vi "CMD tasklist.vi"(8 "error in":errorcluster, 11 "PID":string) -> (0 "error out":errorcluster, 1 "output":string, 2 "tasklist command":string, 3 "Finished":bool)   [LabVIEW 2019, in "PostBuildSupport.lvclass"]
uses:
  PostBuildSupport.lvclass
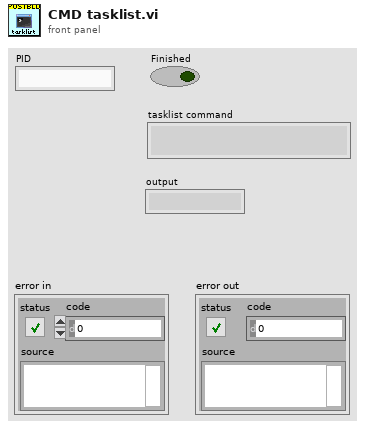
[diagram p1: front panel]
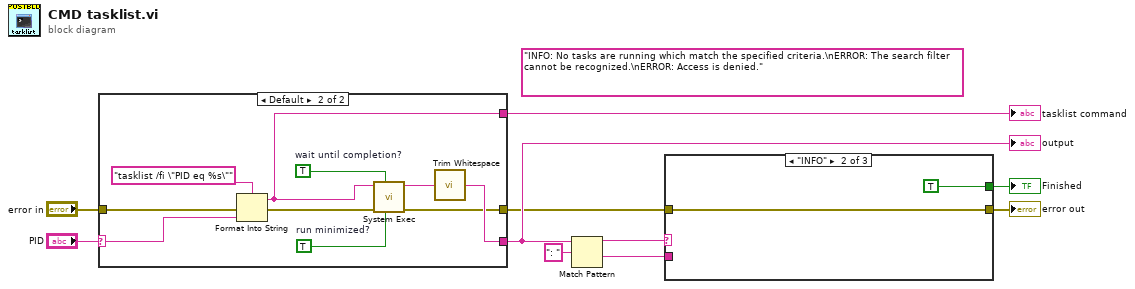
[diagram p0: block diagram]
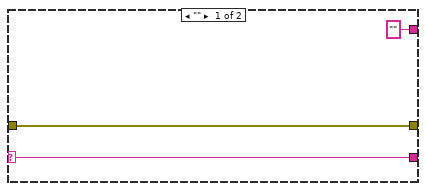
[diagram p2: hidden frame]
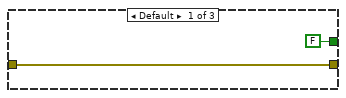
[diagram p3: hidden frame]
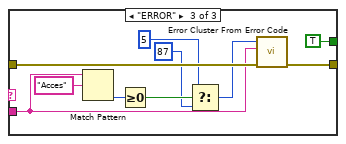
[diagram p4: hidden frame]
diagram:
  (unwired) "INFO: No tasks are running which match the specified criteria.\nERROR: The search filter cannot be recognized.\nERROR: Access is denied." ("x")
  n1 = case shown="Default" "PID" {
    selector: "PID" -> [w13 w20]
    tunnel: [w13 w16] -> w7
    tunnel: "error in" -> [w11 w18]
    tunnel: ["" w15] -> w8
    tunnel: [w11 w14] -> w4
    frame "" {
    }
    frame Default {
      w23 = TRUE  # run minimized?
      w22 = TRUE  # wait until completion?
      n2 = Format Into String(format string="tasklist /fi \"PID eq %s\"" ("command line"), error in=w18, w20) -> (resulting string=w15:string, error out=w17:errorcluster)  [unwired: 1 in]
      n3 = call <vilib>:"System Exec.vi"("run minimized? (F)"=w23, "wait until completion? (T)"=w22, "error in (no error)"=w17, "command line"=w15) -> ("error out"=w14:errorcluster, "standard output"=w19:string)  [unwired: 4 in, 2 out]
      n4 = call <vilib>:"Trim Whitespace.vi"("string"=w19) -> ("trimmed string"=w16:string)  [unwired: 1 in]
    }
  }
  "output" <- w7
  "tasklist command" <- w8
  n5 = Match Pattern(string=w7, regular expression=": ") -> (before substring=w5:string, after substring=w3:string)  [unwired: 1 in, 2 out]
  n6 = case shown="\"INFO\"" w5 {
    tunnel: w4 -> [w25 w27 w37]
    tunnel: w3 -> [_ _ w36]
    tunnel: [w25 w27 w29] -> w1
    tunnel: [FALSE ("Finished") TRUE ("Finished") TRUE ("Finished")] -> w2
    frame Default {
    }
    frame "INFO" {
    }
    frame "ERROR" {
      n7 = Match Pattern(string=w36, regular expression="Acces") -> (offset past match=w34:i32)  [unwired: 1 in, 3 out]
      n8 = Greater Or Equal To 0?(x=w34) -> (x >= 0?=w33:bool)
      n9 = Select(t=5 ("error code (0)"), s=w33, f=87 ("error code (0)")) -> (s? t:f=w31:i32)
      n10 = call <vilib>:"Error Cluster From Error Code.vi"("error in (no error)"=w37, "error message (\"\")"=w36, "error code (0)"=w31) -> ("error out"=w29:errorcluster)  [unwired: 6 in]
    }
  }
  "Finished" <- w2
  "error out" <- w1
